vi "Update Balance Using Account Number.vi"(8 "error in":errorcluster, 10 "New Balance":dbl format="%#.2g", 11 "Account Number":i32) -> (0 "error out":errorcluster, 3 "DB Item":T1 {"Balance" format="%#.2g"})   [LabVIEW 2020, in "Configuration Database.lvlib"]
doc: "Internal Reference holder for Database"
uses:
  Configuration Database.lvlib
  Controls/DB item.ctl
  Controls/FGV Mode.ctl
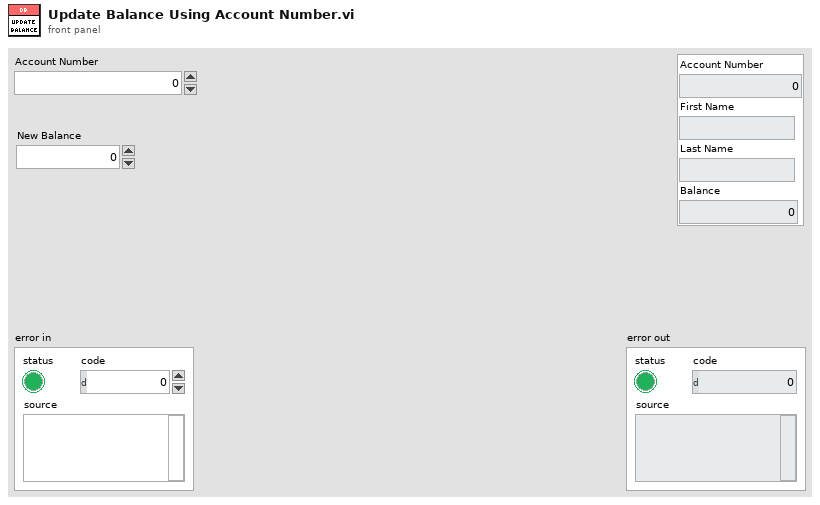
[diagram p1: front panel]
types:
  T1 = typedef "Configuration Database.lvlib/DB item.ctl" = cluster{"Account Number":i32, "First Name":string, "Last Name":string, "Balance":dbl}
  T2 = typedef "Configuration Database.lvlib/FGV Mode.ctl" = enum16{"Initialize", "Get", "Set"}
  T3 = typedef "Configuration Database.lvlib/FGV Data.ctl" = cluster{"CSV File Path":path, "Records":T1[]}
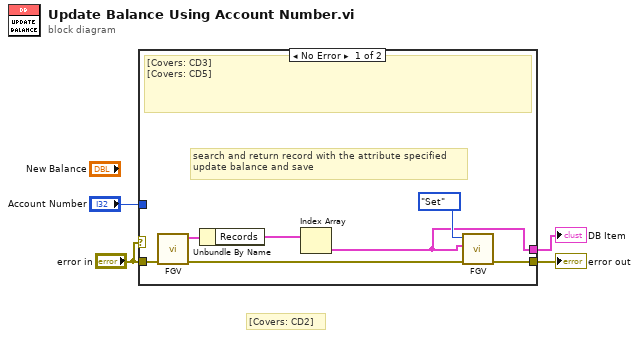
[diagram p0: block diagram]
diagram:
  # "[Covers: CD2]"
  n1 = case shown="No Error" "error in" {
    tunnel: [w7 w12] -> w4
    tunnel: "error in" -> [w11 w12]
    tunnel: [w5 _] -> w2
    tunnel: "Account Number" -> [_ _]
    frame No Error {
      # "search and return record with the attribute specified\nupdate balance and save"
      # "[Covers: CD3]\n[Covers: CD5]"
      n2 = call "FGV.vi"("error in"=w11) -> ("error out"=w8:errorcluster, "Defaults"=w10:T3)  [unwired: 9 in]
      n3 = Unbundle By Name(w10) -> ("Records"=w9:T1[])
      n4 = Index Array(array=w9) -> (element=w5:T1)  [unwired: 1 in]
      n5 = call "FGV.vi"("error in"=w8, "DB Item"=w5, "Mode"=FGV_Mode."Set") -> ("error out"=w7:errorcluster)  [unwired: 7 in, 1 out]
    }
    frame Error {
    }
  }
  "error out" <- w4
  "DB Item" <- w2
